vi "Set Next State.vi"(8 "error in (no error)":errorcluster, 11 "State Machine in":refnum<class "CM_State Machine.lvclass">) -> (0 "error out":errorcluster, 3 "State Machine out":refnum<class "CM_State Machine.lvclass">)   [LabVIEW 2018, in "CM_State Machine.lvclass"]
doc: "Write the next stat to the current state"
uses:
  CM_State Machine.lvclass
  CM_State Machine.lvclass/CM_State Machine.ctl
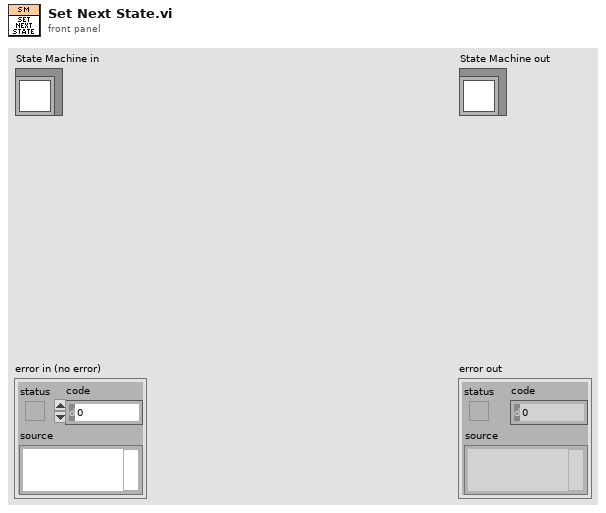
[diagram p1: front panel]
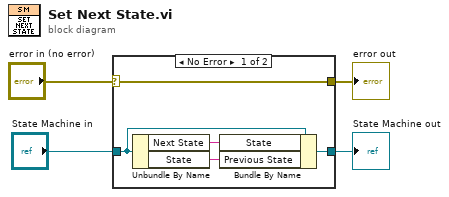
[diagram p0: block diagram]
diagram:
  n1 = case shown="No Error" "error in (no error)" {
    selector: "error in (no error)" -> [w9 w11]
    tunnel: [w9 w11] -> w3
    tunnel: [w8 w10] -> w1
    tunnel: "State Machine in" -> [w7 w10]
    frame No Error {
      n2 = Unbundle By Name(w7) -> ("Next State"=w5:string, "State"=w6:string)
      n3 = Bundle By Name(cluster=w7, "State"=w5, "Previous State"=w6) -> (w8:refnum<class "CM_State Machine.lvclass">)
    }
    frame Error {
    }
  }
  "error out" <- w3
  "State Machine out" <- w1
